vi "GenINI_Build_Read.vi"(8 "error in (no error)":errorcluster, 10 "INI read values":T1[](array[typedef]), 11 "Typedef path":path) -> (0 "error out":errorcluster, 2 "INI read values dup":T1[](array[typedef]), 3 "Typedef path dup":path)   [LabVIEW 2009]
doc: "Build an ini file reader based on the ini file information available."
uses:
  Typedefs/GenINI_Key_Values.ctl
  Typedefs/GenINI_Read_Types.ctl
  <vilib>/Utility/miscctls.llb/LVPointTypeDef.ctl
  <vilib>/Utility/miscctls.llb/LVPositionTypeDef.ctl
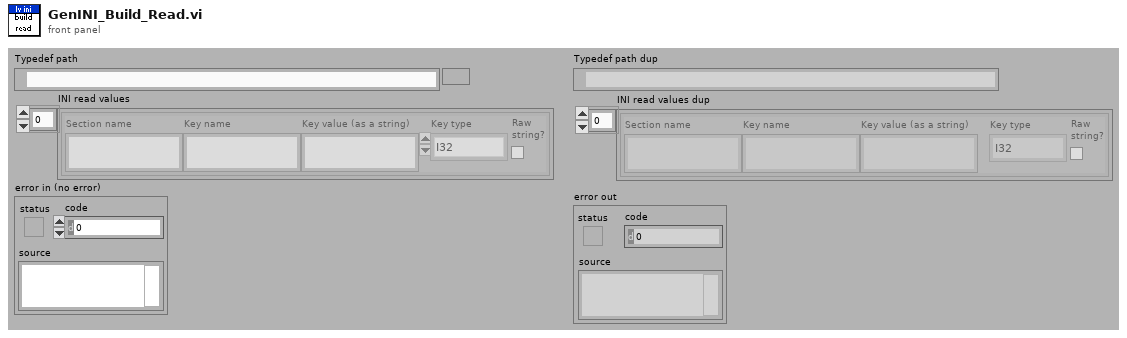
[diagram p1: front panel]
types:
  T1 = typedef "GenINI_Key_Values.ctl" = cluster{"Section name":string, "Key name":string, "Key value (as a string)":string, "Key type":T2, "Raw\nstring?":bool}
  T2 = typedef "GenINI_Read_Types.ctl" = enum16{"Boolean", "Double", "I32", "Path", "String", "U32"}
  T3 = typedef "LVPositionTypeDef.ctl" = cluster{"Left":i32, "Top":i32}
  T4 = typedef "LVPointTypeDef.ctl" = cluster{"Horizontal":i16, "Vertical":i16}
  T5 = cluster{"left":i16, "top":i16, "right":i16, "bottom":i16}
  T6 = enum32{"invalid VI type", "Standard VI", "Control VI", "Global VI", "Polymorphic VI", "Configuration VI", "SubSystem", "Facade VI", "Method VI", "Statechart Diagram VI"}
  T7 = typedef "LVRectTypeDef.ctl" = cluster{"left":i16, "top":i16, "right":i16, "bottom":i16}
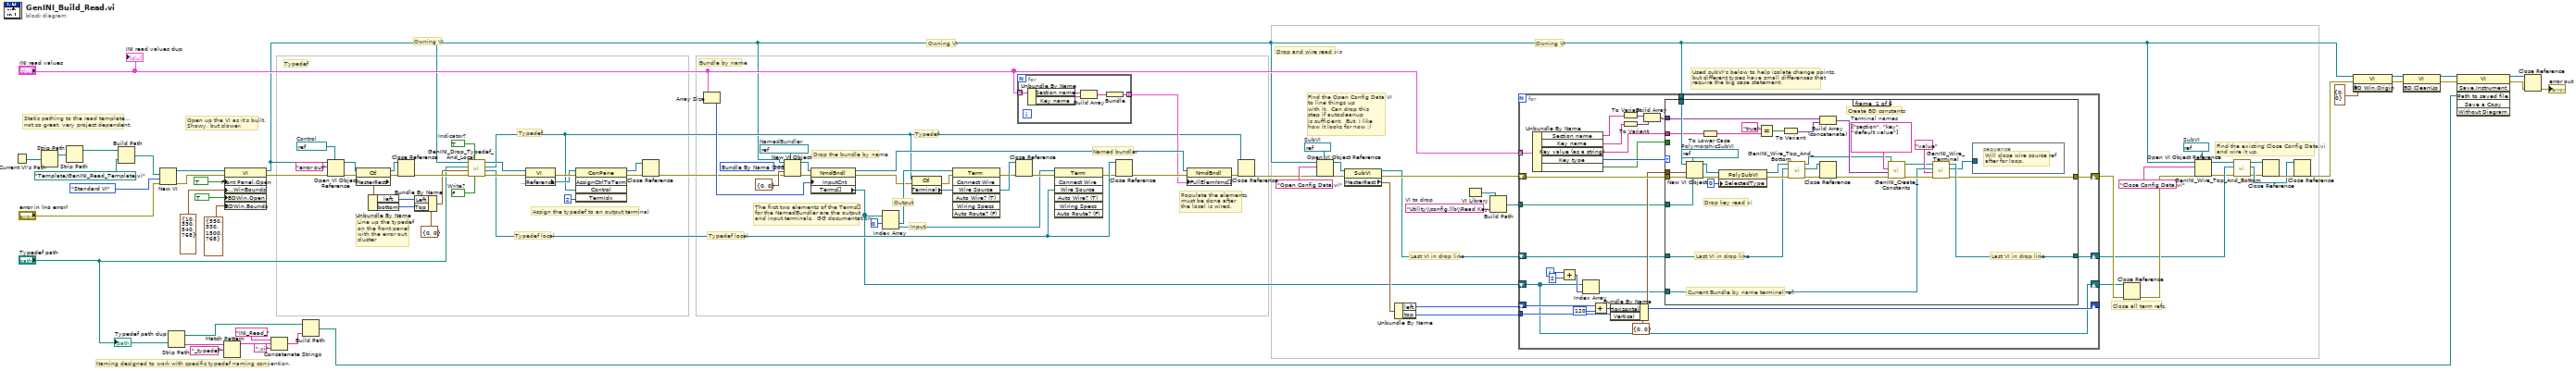
[diagram p0: block diagram]
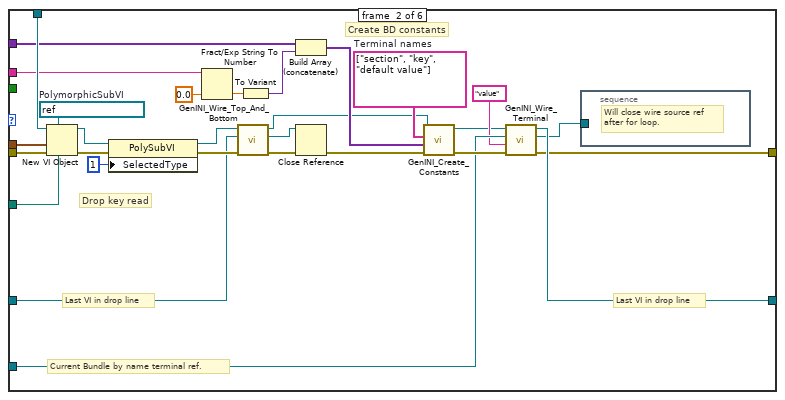
[diagram p2: hidden frame]
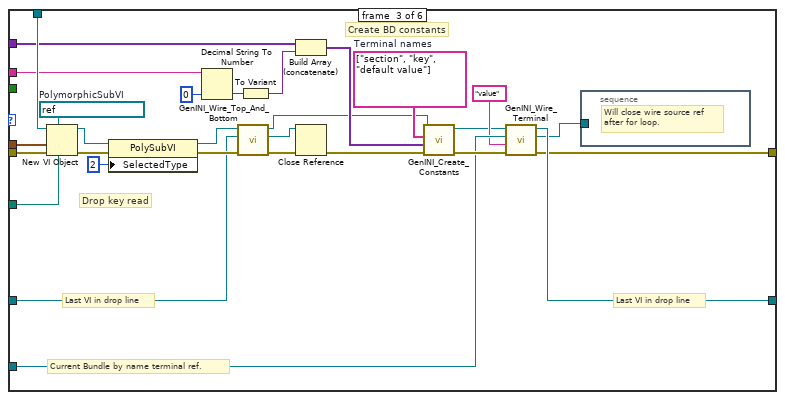
[diagram p3: hidden frame]
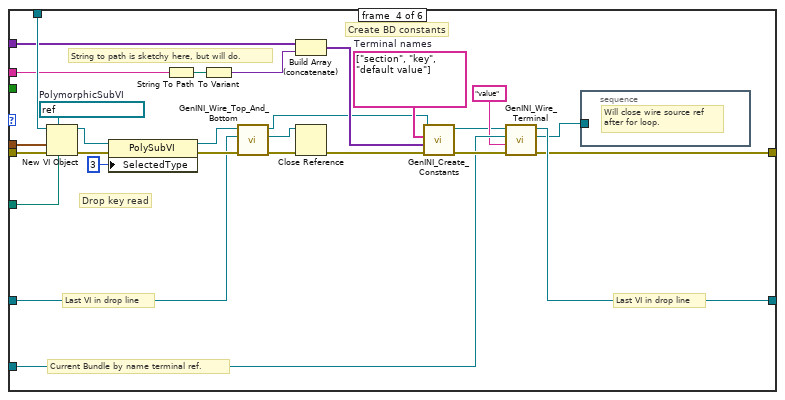
[diagram p4: hidden frame]
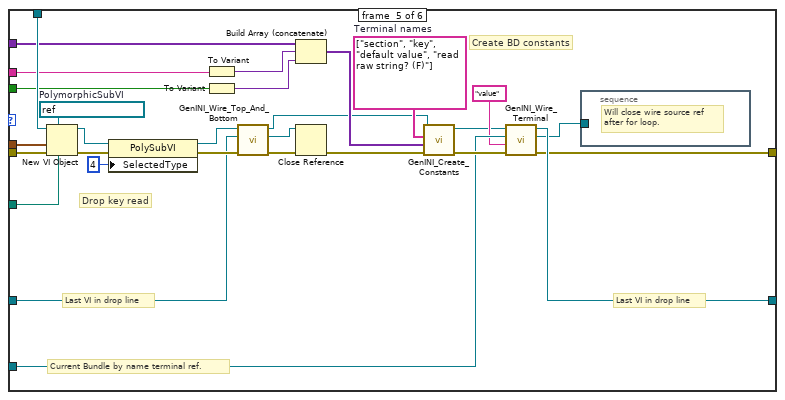
[diagram p5: hidden frame]
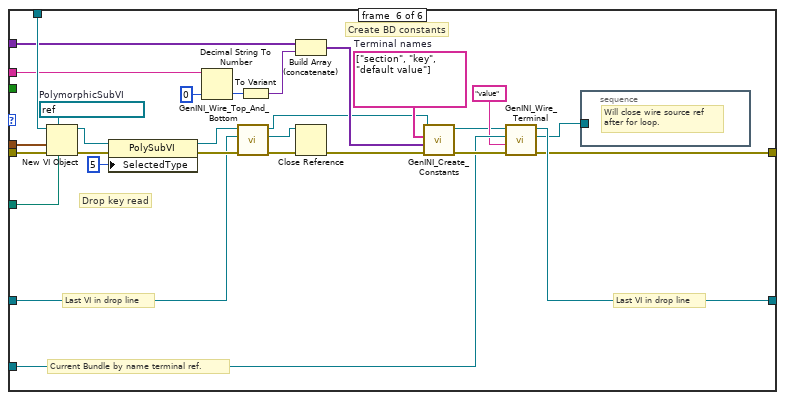
[diagram p6: hidden frame]
diagram:
  w29 = refnum<vi> refnum  # Control
  w57 = FALSE  # Write?
  w69 = TRUE  # Indicator?
  w78 = "Utility\\config.llb\\Read Key.vi"  # VI to drop
  w83 = refnum<vi> refnum  # SubVI
  w87 = refnum<vi> refnum  # SubVI
  w89 = refnum<vi> refnum  # NamedBundler
  w90 = 2057 items=[".NET Container"=2125, ".NET Refnum"=3441, "2D Picture"=3508, "3D Picture"=23776, "Absolute Value"=1054, "Access Rights"=1412, "ActiveX Container"=2072, "Add"=3915, "Add 1"=1050, "Add Array Elements"=1903, "Agitator"=3831, "AllSpoll"=1960, "Always Copy"=2400, "And"=1061, "And Array Elements"=1911, "Append True/False String"=1511, "Application Refnum"=3412, "Array"=21608, "Array 1"=3300, "Array Constant"=2070, "Array Interface Control"=23777, "Array Max & Min"=1907, "Array Size"=1809, "Array Subset"=2044, "Array To Cluster"=1168, "Array To Spreadsheet String"=1540, "Array of Strings to Path"=1422, "Atmospheric Tank"=3070, "Atmospheric Tank 1"=21751, "Automation Close"=8001, "Automation Open"=8000, "Automation Refnum"=3410, "Avogadro Constant (1/mol)"=23520, "Base 10 Logarithm Of e"=23512, "Bin"=3073, "Bin 1"=21755, "Bitpack to Array"=3135, "Blocking Variable Read"=23786, "Blocking Variable Write"=23789, "Bluetooth Close Connection"=9148, "Bluetooth Create Listener"=9151, "Bluetooth Discover"=9152, "Bluetooth Network Connection Refnum"=3468, "Bluetooth Open Connection"=9153, "Bluetooth Read"=9149, "Bluetooth Wait On Listener"=9147, "Bluetooth Write"=9150, "Boolean Array To Number"=1815, "Boolean To (0,1)"=1167, "Build Array"=2041, "Build Cluster Array"=2047, "Build Matrix"=8500, "Build Path"=1419, "Build Waveform"=2066, "Bundle"=2049, "Bundle By Name"=2057, "Byte Array To String"=1609, "Byte Stream File Refnum"=3408, "CAN Channel"=21966, "CAN Channel 1"=3340, "CAN Channel 2"=2124, "CAN Channel 3"=21817, "CAN Interface"=3339, "CAN Interface 1"=21815, "CAN Interface 2"=2123, "CAN Interface 3"=21964, "CAN Task"=3470, "CAN Task 1"=3471, "CAN Task 2"=21963, "CAN Task 3"=21789, "CPU Information"=24130, "Call By Reference Node"=3901, "Call Chain"=1999, "Call Library Function Node"=2062, "Call Parent Method"=2354, "Cancel Button"=21739, "Cancel Notification"=9107, "Carriage Return Constant"=23500, "Case Structure"=2001, "Cast Unit Bases"=1079, "Check Valve"=3833, "Checkbox"=3117, "Class Specifier Constant"=2094, "Classic Radio Buttons"=22003, "Clear Fixed-Point Overflow Status"=5562, "Close File"=1405, "Close File 1"=8052, "Close Reference"=8011, "Close Variable Connection"=23783, "Cluster"=3400, "Cluster 1"=21607, "Cluster Constant"=2071, "Cluster To Array"=1169, "Code Interface Node"=2050, "Coerce To Type"=2402, "Color Box"=3013, "Color Box Constant"=2120, "Color Box Thin Border"=2905, "Color Ramp"=3022, "Combo Box"=21604, "Combo Box 1"=3304, "Combo Box Constant"=2088, "Complex Conjugate"=1048, "Complex To Polar"=1045, "Complex To Re/Im"=1044, "Compound Arithmetic"=2200, "Compressor"=3832, "Concatenate Strings"=2040, "Conditional Disable Structure"=2064, "Constructor Node"=3904, "Control & Simulation Loop"=2099, "Control Help Window"=1353, "Control Online Help"=1355, "Control Refnum"=3419, "Convert Unit"=2059, "Conveyer"=3827, "Copy"=1416, "Copy 1"=8053, "Cosecant"=1204, "Cosine"=1201, "Cotangent"=1205, "Create Folder"=8055, "Create User Event"=2073, "Current Processor ID"=24131, "Current VI's Menubar"=9000, "Current VI's Path"=1426, "DAQmx Analog Trigger Source"=3336, "DAQmx Analog Trigger Source 1"=2119, "DAQmx Analog Trigger Source 2"=21951, "DAQmx Analog Trigger Source 3"=21774, "DAQmx Device Name"=21773, "DAQmx Device Name 1"=21950, "DAQmx Device Name 2"=2093, "DAQmx Device Name 3"=3318, "DAQmx Global Channel"=3443, "DAQmx Global Channel 1"=21770, "DAQmx Global Channel 2"=21957, "DAQmx Global Channel 3"=3430, "DAQmx Physical Channel"=3335, "DAQmx Physical Channel 1"=21954, "DAQmx Physical Channel 2"=2118, "DAQmx Physical Channel 3"=21777, "DAQmx Scale Name"=21952, "DAQmx Scale Name 1"=21775, "DAQmx Scale Name 2"=3317, "DAQmx Scale Name 3"=2116, "DAQmx Switch"=21953, "DAQmx Switch 1"=3337, "DAQmx Switch 2"=2121, "DAQmx Switch 3"=21776, "DAQmx Task Name"=3442, "DAQmx Task Name 1"=3434, "DAQmx Task Name 2"=21959, "DAQmx Task Name 3"=21778, "DAQmx Terminal"=21955, "DAQmx Terminal 1"=2117, "DAQmx Terminal 2"=21781, "DAQmx Terminal 3"=3319, "Data Cache Size"=24132, "Data Log File Refnum"=3402, "DataSocket Close"=1085, "DataSocket Open"=1084, "DataSocket Read"=1086, "DataSocket Refnum"=3417, "DataSocket Write"=1087, "Date/Time To Seconds"=1308, "Decimal Digit?"=1119, "Decimal String To Number"=1184, "Decimate 1D Array"=2046, "DecomposeArray"=2412, "DecomposeLockDataValRef"=2406, "DecomposeVariant"=2404, "Decrement"=1058, "Default Directory"=1427, "Delete"=8056, "Delete 1"=1417, "Delete Data Value Reference"=2409, "Delete From Array"=3912, "Delete Menu Items"=9004, "Delete Variant Attribute"=8206, "Delete Waveform Attribute"=8209, "Deny Access"=8057, "Dequeue Element"=9113, "Destroy User Event"=2075, "DevClear"=1961, "DevClearList"=1962, "Device Control/Status"=1433, "Device Refnum"=3405, "Diagram Disable Structure"=2054, "Dial"=3050, "Dial 1"=21732, "Digital Data"=3210, "Digital Data 1"=21216, "Digital Waveform Graph"=21718, "Digital Waveform Graph 1"=3511, "Direct Variable Read"=23785, "Direct Variable Write"=23788, "Divide"=1053, "Divide 1"=3918, "Dlg CheckBox"=21924, "Dlg Horiz Scrollbar"=21905, "Dlg Numeric"=2100, "Dlg Numeric 2"=3006, "Dlg String"=2110, "Dlg Vert Scrollbar"=21906, "Down Arrow"=3824, "Down Bow Valve"=3707, "Down Bow Valve 1"=21767, "Down Bow Valve 2"=3807, "Down Rect Valve"=21766, "Down Rect Valve 1"=3706, "Down Rect Valve 2"=3806, "Down Tee"=3818, "Down Tee 1"=3718, "EOF"=1410, "Elementary Charge (C)"=23517, "Empty Array?"=23063, "Empty Path Constant"=23523, "Empty String Constant"=23503, "Empty String/Path?"=1112, "Enable Menu Tracking"=9002, "EnableLocal"=1963, "EnableRemote"=1964, "End of Line Constant"=23525, "Enqueue Element"=9111, "Enqueue Element At Opposite End"=9129, "Enum"=3023, "Enum 1"=21605, "Enum Constant"=2090, "Equal To 0?"=1113, "Equal?"=1102, "Error Ring Constant"=2039, "Event Callback Refnum"=3435, "Event Data Node"=2102, "Event Structure"=2052, "Exchanger"=3828, "Exclusive Or"=1063, "Exponential"=1211, "Exponential (Arg) -1"=1222, "Expression Node"=2201, "FIFO Refnum"=3474, "False Constant"=2006, "Feedback Node, Feedback Node 1"=2353, "FieldPoint IO Point"=21784, "FieldPoint IO Point 1"=3440, "FieldPoint IO Point 2"=3439, "File Dialog"=8058, "File Dialog 1"=8081, "File Path Control"=21730, "File Path Control 1"=3203, "File Path Indicator"=21731, "File Path Indicator 1"=3204, "File/Directory Info"=1413, "File/Directory Info 1"=8082, "FindLstn"=1965, "FindRQS"=1966, "First Call?"=1083, "Fixed-Point Overflow?"=5565, "Fixed-Point to Integer Cast"=5566, "Flat Box"=3602, "Flat Circle"=3605, "Flat Down Triangle"=3623, "Flat Frame"=3608, "Flat Left Triangle"=3620, "Flat Right Triangle"=3621, "Flat Round Button"=3102, "Flat Rounded Box"=3611, "Flat Sequence Structure"=2069, "Flat Square Button"=3103, "Flat Up Triangle"=3622, "Flatten To String"=1164, "Flatten To XML"=8400, "Flattened String To Variant"=8202, "Floating Point Equal?"=23064, "Flush File"=8059, "Flush File 1"=1406, "Flush Queue"=9114, "For Loop"=2002, "Fork"=2194, "Format Date/Time String"=8100, "Format Into File"=2083, "Format Into String"=2081, "Format Value"=1512, "Formula Node"=2004, "Fract/Exp String To Number"=1187, "Framed Color Box"=21019, "Framed Color Box 1"=3008, "Free Label"=2321, "Furnace"=3829, "GPIB Clear"=1954, "GPIB Initialization"=1957, "GPIB Misc"=1956, "GPIB Read"=1951, "GPIB Serial Poll"=1955, "GPIB Status"=1959, "GPIB Trigger"=1953, "GPIB Wait"=1958, "GPIB Write"=1950, "Gauge"=21009, "Gauge 1"=3040, "Generate Front Panel Activity"=1329, "Generate Occurrence"=1700, "Generate User Event"=2074, "Generate User-Defined Trace Event"=2250, "Get Datalog Position"=8061, "Get Date/Time In Seconds"=1303, "Get Date/Time String"=1600, "Get Drag Drop Data"=9154, "Get File Position"=8062, "Get File Size"=8063, "Get Fixed-Point Components"=11163, "Get Help Window Status"=1354, "Get Matrix Diagonal"=8501, "Get Matrix Elements"=8502, "Get Menu Item Info"=9005, "Get Menu Selection"=9001, "Get Menu Short Cut Info"=9007, "Get Notifier Status"=9103, "Get Number of Records"=8064, "Get Permissions"=8065, "Get Queue Status"=9110, "Get Submatrix"=8503, "Get Type and Creator"=8066, "Get Variant Attribute"=8205, "Get Volume Info"=8067, "Get Waveform Attribute"=8208, "Get Waveform Components"=2067, "Global Variable"=2060, "Gravitational Constant (N m2/kg2)"=23519, "Greater Or Equal To 0?"=1114, "Greater Or Equal?"=1103, "Greater Than 0?"=1117, "Greater?"=1110, "Handle Peek"=1604, "Handle Poke"=1605, "Hex Digit?"=1123, "Hexadecimal String To Number"=1185, "Hopper"=21754, "Hopper 1"=3072, "Horiz Line"=3821, "Horiz Pipe"=3710, "Horiz Pipe 1"=3810, "Horizontal Button Box"=3636, "Horizontal Fill Slide"=3012, "Horizontal Fill Slide 1"=21100, "Horizontal Graduated Bar"=21106, "Horizontal Pointer Slide"=21101, "Horizontal Pointer Slide 1"=3011, "Horizontal Progress Bar"=21102, "Horizontal Scrollbar"=21110, "Horizontal Slide"=3010, "Horizontal Slide Switch"=3114, "Horizontal Smooth Box"=3633, "Horizontal Splitter Bar"=21861, "Horizontal Splitter Bar (Classic)"=21863, "Horizontal Splitter Bar (System)"=21865, "Horizontal Switch"=3108, "Horizontal Tank"=3071, "Horizontal Toggle Switch"=3110, "Horizontal Toggle Switch 1"=21700, "Hyperbolic Cosecant"=23053, "Hyperbolic Cosine"=1215, "Hyperbolic Cotangent"=23055, "Hyperbolic Secant"=23054, "Hyperbolic Sine"=1214, "Hyperbolic Tangent"=1216, "IMAQ Session"=3415, "IP To String"=1710, "IVI Delete Session"=8103, "IVI Logical Name"=3420, "IVI Logical Name 1"=3414, "IVI Logical Name 2"=21736, "IVI New Session"=8102, "Implies"=1080, "In Place Element Structure"=2360, "In Range and Coerce"=1127, "Include Fixed-Point Overflow Status"=5564, "Increment"=1057, "Index & Bundle Cluster Array"=2056, "Index Array"=2042, "Index String Array"=1531, "Initialize Array"=2053, "Inline C Node"=2104, "Insert Into Array"=3911, "Insert Menu Items"=9003, "Integer to Fixed-Point Cast"=5567, "Intensity Chart"=21719, "Intensity Chart 1"=3509, "Intensity Graph"=21720, "Intensity Graph 1"=3510, "Interleave 1D Arrays"=2045, "Interpolate 1D Array"=1905, "Inverse Cosecant"=23050, "Inverse Cosine"=1207, "Inverse Cotangent"=23052, "Inverse Hyperbolic Cosecant"=23056, "Inverse Hyperbolic Cosine"=1218, "Inverse Hyperbolic Cotangent"=23058, "Inverse Hyperbolic Secant"=23057, "Inverse Hyperbolic Sine"=1217, "Inverse Hyperbolic Tangent"=1219, "Inverse Secant"=23051, "Inverse Sine"=1206, "Inverse Tangent"=1208, "Inverse Tangent (2 Input)"=1228, "Invoke Node"=3900, "IrDA Close Connection"=9144, "IrDA Create Listener"=9140, "IrDA Discover"=9141, "IrDA Network Connection Refnum"=3450, "IrDA Open Connection"=9142, "IrDA Read"=9145, "IrDA Wait On Listener"=9143, "IrDA Write"=9146, "Join"=2195, "Join Numbers"=1171, "Junction"=2197, "Knob"=21000, "Knob 1"=3005, "LED Button"=3116, "LabVIEW Object"=3457, "Label"=21960, "Labeled Oblong Button"=3125, "Labeled Rectangular Button"=3124, "Labeled Round Button"=3122, "Labeled Square Button"=3123, "Leak Variant Value Reference"=2410, "Left Arrow"=3826, "Left Bow Valve"=3701, "Left Bow Valve 1"=3801, "Left Bow Valve 2"=21761, "Left Down Elbow"=3711, "Left Down Elbow 1"=3811, "Left Pump"=3713, "Left Pump 1"=3813, "Left Rect Valve"=3700, "Left Rect Valve 1"=21760, "Left Rect Valve 2"=3800, "Left Tee"=3709, "Left Tee 1"=3809, "Left Up Elbow"=3808, "Left Up Elbow 1"=3708, "Less Or Equal To 0?"=1115, "Less Or Equal?"=1104, "Less Than 0?"=1118, "Less?"=1111, "Lexical Class"=1126, "Line Feed Constant"=23501, "List Directory"=1418, "List Folder"=8083, "Listbox"=21792, "Listbox 1"=21806, "Listbox Symbol Ring Constant"=2038, "Local Variable"=2061, "Lock Range"=1411, "Logarithm Base 10"=1210, "Logarithm Base 2"=1225, "Logarithm Base X"=1224, "Logical Shift"=1081, "Lossy Enqueue Element"=9130, "Lowered Rounded Box"=3638, "MATLAB script"=9020, "Machine Epsilon"=23528, "MakeAddr"=1967, "Mantissa & Exponent"=1150, "Match First String"=1532, "Match Pattern"=1535, "Match True/False String"=1533, "MathScript Call By Reference Node"=3906, "MathScript Node"=2357, "Matrix Size"=8507, "Max & Min"=1108, "Menu Refnum"=3413, "Menu Ring"=3018, "Menu Ring 1"=21600, "Menu-Popup Ring"=3017, "Merge Signals"=2350, "Meter"=21008, "Meter 1"=3030, "Mixed Signal Graph"=21721, "Molar Gas Constant (J/(mol K))"=23522, "Motion Resource"=21787, "Motion Resource 1"=3448, "Motion Resource 2"=3449, "Motor"=3720, "Motor 1"=3820, "Move"=1415, "Move 1"=8068, "Multi-Segment Pipe"=23780, "Multicolumn Listbox"=21799, "Multicolumn Listbox 1"=21791, "Multiple Selection Listbox"=3208, "Multiply"=1052, "Multiply 1"=3917, "Multiply Array Elements"=1904, "Multirate Structure"=2199, "Natural Logarithm"=1209, "Natural Logarithm (Arg +1)"=1221, "Natural Logarithm Base"=23510, "Natural Logarithm Of 10"=23513, "Natural Logarithm Of 2"=23514, "Natural Logarithm Of Pi"=23508, "Negate"=1069, "Negative Infinity"=23509, "New Data Value Reference"=2408, "New Directory"=1402, "New File"=1404, "New VI"=8014, "New VI Object"=8015, "Not"=1064, "Not A Number/Path/Refnum?"=1128, "Not A Path Constant"=23524, "Not And"=1071, "Not Equal To 0?"=1116, "Not Equal?"=1105, "Not Exclusive Or"=1073, "Not Or"=1072, "Not a Refnum Constant"=23526, "Not a Shared Variable"=23527, "Notifier Refnum"=3423, "Number To Boolean Array"=1814, "Number To Decimal String"=1180, "Number To Engineering String"=1183, "Number To Exponential String"=1505, "Number To Fractional String"=1506, "Number To Hexadecimal String"=1181, "Number To Octal String"=1182, "Number of Cache Levels"=24133, "Numeric Constant"=2005, "Numeric Control"=3000, "Numeric Control 1"=21003, "Numeric Indicator"=3001, "Numeric Indicator 1"=21004, "OK Button"=21738, "OLE Variant"=3150, "Obtain Notifier"=9101, "Obtain Queue"=9108, "Occurrence Refnum"=3406, "Octal Digit?"=1129, "Octal String To Number"=1186, "Old VISA Open"=1921, "One Button Dialog"=1340, "Open Application Reference"=8012, "Open Device"=1430, "Open File"=1403, "Open Tank"=21752, "Open Tank 1"=3074, "Open VI Object Reference"=8013, "Open VI Reference"=8010, "Open Variable Connection"=23779, "Open Variable Connection in Background"=23791, "Open and Verify Variable Connection"=23790, "Open/Create/Replace Datalog"=8054, "Open/Create/Replace File"=8050, "Or"=1062, "Or Array Elements"=1910, "PPoll"=1969, "PPollConfig"=1970, "PPollUnconfig"=1971, "Package Matrix"=23001, "PassControl"=1968, "Path Constant"=2009, "Path To String"=1077, "Path Type"=1421, "Path to Array of Strings"=1423, "Pi"=23504, "Pi Divided By 2"=23506, "Pi Multiplied By 2"=23505, "Pick Line"=1510, "Pict Ring"=21602, "Pict Ring 1"=3015, "PixMap"=3505, "PixMap (Do not touch it!!)"=3507, "Planck's Constant (J/Hz)"=23516, "Platform Flat Square Button"=3134, "Plug-In Control"=21820, "Polar To Complex"=1047, "Polar To Re/Im"=23061, "Positive Infinity"=23515, "Power Of 10"=1212, "Power Of 2"=1223, "Power Of X"=1213, "Preserve Run-Time Class"=8018, "Pressure Tank"=3075, "Pressure Tank 1"=21753, "Preview Queue Element"=9112, "Printable?"=1124, "Property Node"=1920, "Pulldown Menu Ring"=3061, "Push Button"=21001, "Queue Refnum"=3424, "Quit LabVIEW"=1352, "Quotient & Remainder"=1056, "RT FIFO Create"=24000, "RT FIFO Delete"=24003, "RT FIFO Read"=24001, "RT FIFO Write"=24002, "Radio Buttons"=22001, "Raised Box"=3600, "Raised Box 1"=3637, "Raised Circle"=3603, "Raised Down Triangle"=3615, "Raised Frame"=3606, "Raised Left Triangle"=3612, "Raised Right Triangle"=3613, "Raised Rounded Box"=3609, "Raised Up Triangle"=3614, "Random Number (0-1)"=1070, "RcvRespMsg"=1972, "Re/Im To Complex"=1046, "Re/Im To Polar"=23060, "Read Datalog"=8069, "Read Device"=1432, "Read File"=1407, "Read Variable"=23781, "Read from Binary File"=8051, "Read from Text File"=8070, "ReadStatus"=1973, "Receive"=1974, "ReceiveSetup"=1975, "Recessed Box"=3601, "Recessed Circle"=3604, "Recessed Down Triangle"=3619, "Recessed Frame"=3607, "Recessed Left Triangle"=3616, "Recessed Menu Ring"=3019, "Recessed Right Triangle"=3617, "Recessed Rounded Box"=3610, "Recessed Up Triangle"=3618, "Reciprocal"=1059, "Reciprocal Of Pi"=23507, "Reciprocal Of e"=23511, "RecomposeArray"=2403, "RecomposeUnlockDataValRef"=2407, "RecomposeVariant"=2405, "Rectangular Stop Button"=3128, "Refnum to Path"=1424, "Refnum to Session"=2306, "Region"=2196, "Register Event Callback"=2078, "Register For Events"=2065, "Register Session"=2319, "Release Notifier"=9102, "Release Queue"=9109, "Remove Fixed-Point Overflow Status"=5563, "Replace Array Subset"=3910, "Replace Substring"=3913, "Request Deallocation"=1610, "ResetSys"=1976, "Reshape Array"=2055, "Resize Matrix"=8508, "Reverse 1D Array"=1900, "Reverse String"=1537, "Right Arrow"=3825, "Right Bow Valve"=21765, "Right Bow Valve 1"=3705, "Right Bow Valve 2"=3805, "Right Down Elbow"=3817, "Right Down Elbow 1"=3717, "Right Pump"=3719, "Right Pump 1"=3819, "Right Rect Valve"=3804, "Right Rect Valve 1"=3704, "Right Rect Valve 2"=21764, "Right Tee"=3715, "Right Tee 1"=3815, "Right Up Elbow"=3814, "Right Up Elbow 1"=3714, "Ring Constant"=2008, "Rocker"=21002, "Rotary Feeder"=3830, "Rotate"=1082, "Rotate 1D Array"=1906, "Rotate Left With Carry"=1606, "Rotate Right With Carry"=1607, "Rotate String"=1536, "Round Button"=3100, "Round LED"=3120, "Round LED 1"=21012, "Round Light"=3104, "Round Push Button"=3112, "Round Push Button 2"=3118, "Round Radio Button"=3106, "Round Stop Button"=3127, "Round To Nearest"=1055, "Round Toward +Infinity"=1076, "Round Toward -Infinity"=1075, "Rydberg Constant (1/m)"=23521, "Scale By Power Of 2"=1074, "Scan From File"=2082, "Scan From String"=2080, "Scan String For Tokens"=8101, "Scan Value"=1534, "Scanned Variable Read"=23784, "Scanned Variable Write"=23787, "Search 1D Array"=1901, "Search and Replace String"=3914, "Search/Split String"=1538, "Secant"=1203, "Seconds To Date/Time"=1309, "Seek"=1409, "Select"=1516, "Send"=1977, "Send Notification"=9104, "SendCmds"=1978, "SendDataBytes"=1979, "SendIFC"=1980, "SendLLO"=1982, "SendList"=1981, "SendSetup"=1983, "Session to Refnum"=2307, "Set Datalog Position"=8072, "Set File Position"=8073, "Set File Size"=8074, "Set Matrix Diagonal"=8504, "Set Matrix Elements"=8505, "Set Menu Item Info"=9006, "Set Number of Records"=8075, "Set Occurrence"=1702, "Set Permissions"=8076, "Set Submatrix"=8506, "Set Type and Creator"=8077, "Set Variant Attribute"=8204, "Set Waveform Attribute"=8207, "SetRWLS"=1984, "SetTimeOut"=1985, "Shared Variable"=23778, "Shared Variable Constant"=3473, "Shared Variable Control"=3472, "Shared Variable Control 1"=21814, "Shared Variable to String"=1831, "Sign"=1049, "Simple Horizontal Slide"=3003, "Simple Numeric"=3029, "Simple Numeric 1"=2900, "Simple String"=2115, "Simple Vertical Slide"=3002, "Sinc"=1227, "Sine"=1200, "Sine & Cosine"=1220, "Size Handle"=1603, "Slide Switch"=21011, "Sort 1D Array"=1120, "Sort Array of String, Sort Array of String 1"=23065, "Speed Of Light In Vacuum (m/sec)"=23518, "Split 1D Array"=1908, "Split Button"=21020, "Split Number"=1170, "Split Signals"=2351, "Spreadsheet String To Array"=1539, "Square"=23059, "Square Button"=3101, "Square LED"=3121, "Square LED 1"=21013, "Square Light"=3105, "Square Push Button"=3113, "Square Push Button 2"=3119, "Square Radio Button"=3107, "Square Root"=1060, "Stacked Sequence Structure"=2000, "State"=2198, "State Diagram"=2051, "Static VI Reference"=2084, "Stop"=1350, "Stop Button"=21230, "String Constant"=2007, "String Control"=3200, "String Control 1"=21701, "String Indicator"=3201, "String Indicator 1"=21702, "String Length"=1502, "String Subset"=1503, "String To Byte Array"=1608, "String To IP"=1711, "String To Path"=1078, "String to Shared Variable"=1830, "Strip Path"=1420, "SubPanel"=21810, "SubPanel (Classic)"=21811, "SubPanel (System)"=21823, "Subtract"=1051, "Subtract 1"=3916, "Swap Bytes"=1162, "Swap Values"=2401, "Swap Vector Element"=1912, "Swap Words"=1163, "System Button"=3130, "System Cancel Button"=3131, "System Checkbox"=3132, "System Chiseled Line"=3632, "System Colored Rectangle"=3625, "System Combo Box"=21917, "System Enum"=3062, "System Horizontal Pointer Slide"=21902, "System Horizontal Progress Bar"=21910, "System Horizontal Slide"=21904, "System Label"=21961, "System Listbox"=21805, "System Mixed Checkbox"=21333, "System Multicolumn Listbox"=21798, "System Numeric"=21919, "System Path Control"=21922, "System Pict Ring"=21925, "System Radio Button"=3133, "System Radio Buttons"=22002, "System Recessed Frame"=3624, "System Ring"=3060, "System Spin Control"=21900, "System String"=21920, "System Tab Control"=3331, "System Table"=21797, "System Time Stamp"=21967, "System Tree"=21794, "System Vertical Pointer Slide"=21901, "System Vertical Progress Bar"=21909, "System Vertical Slide"=21903, "TCP Close Connection"=1713, "TCP Create Listener"=1717, "TCP Flattened Read"=1718, "TCP Flattened Write"=1719, "TCP Flex Read"=1720, "TCP Flex Write"=1721, "TCP Network Connection Refnum"=3407, "TCP Open Connection"=1715, "TCP Read"=1716, "TCP Wait On Listener"=1712, "TCP Write"=1714, "TDMS Close"=24113, "TDMS Defragment"=24119, "TDMS File"=3477, "TDMS Flush"=24117, "TDMS Get Properties"=24115, "TDMS List Contents"=24116, "TDMS Open"=24112, "TDMS Read"=24111, "TDMS Refnum To File ID"=24120, "TDMS Set Properties"=24114, "TDMS Write"=24110, "TDMS Write IP"=24118, "Tab Constant"=23502, "Tab Control"=3330, "Tab Control 1"=3332, "Table"=21796, "Table 1"=21790, "Tag Attribute Ring"=2063, "Tangent"=1202, "Tank"=21006, "Tank 1"=3020, "Temporary Directory"=1435, "TestSRQ"=1986, "TestSys"=1987, "Text & Pict Ring"=21603, "Text & Pict Ring 1"=3016, "Text Button"=21015, "Text Ring"=21601, "Text Ring 1"=3014, "Text to UTF-8"=23066, "Thermometer"=21007, "Thermometer 1"=3021, "Thick Chiseled Line"=3630, "Thick Line"=3629, "Thick Line with Arrow"=3631, "Thick Lowered Box"=3635, "Thin Chiseled Line"=3627, "Thin Line"=3626, "Thin Line with Arrow"=3628, "Threshold 1D Array"=1909, "Tick Count (ms)"=1300, "Time Stamp Constant"=2068, "Time Stamp Control"=21913, "Time Stamp Control 1"=5555, "Time Stamp Indicator"=21914, "Time Stamp Indicator 1"=5556, "Timed Loop"=5570, "Timed Sequence"=5573, "To Byte Integer"=1140, "To Double Precision Complex"=1152, "To Double Precision Float"=1147, "To Extended Precision Complex"=1154, "To Extended Precision Float"=1149, "To Fixed-Point"=5561, "To Long Integer"=1142, "To Lower Case"=1189, "To More Generic Class"=8017, "To More Specific Class"=8016, "To OLE Variant"=8002, "To Probe String"=2413, "To Quad Integer"=1155, "To Single Precision Complex"=1151, "To Single Precision Float"=1146, "To Time Stamp"=5560, "To Unsigned Byte Integer"=1143, "To Unsigned Long Integer"=1145, "To Unsigned Quad Integer"=1156, "To Unsigned Word Integer"=1144, "To Upper Case"=1188, "To Variant"=8201, "To Word Integer"=1141, "Traditional DAQ Channel"=21733, "Traditional DAQ Channel 1"=2085, "Traditional DAQ Channel 2"=3320, "Transpose 1D Array"=23068, "Transpose 2D Array"=1902, "Transpose Matrix"=8509, "Tree"=21819, "Tree 1"=21793, "Trigger"=1988, "TriggerList"=1989, "Two Button Dialog"=1341, "Type Cast"=1166, "Type and Creator"=1434, "UDP Close"=1726, "UDP Multicast Open"=1727, "UDP Network Connection Refnum"=3418, "UDP Open"=1723, "UDP Read"=1724, "UDP Write"=1725, "UTF-8 to Text"=23067, "Unbitpack from Array"=3136, "Unbundle"=2048, "Unbundle By Name"=2058, "Unflatten From String"=1165, "Unflatten From XML"=8401, "Unleak Variant Value Reference"=2411, "Unpackage Matrix"=23000, "Unregister For Events"=2076, "Unregister Session"=2320, "Up Arrow"=3823, "Up Bow Valve"=3703, "Up Bow Valve 1"=3803, "Up Bow Valve 2"=21763, "Up Rect Valve"=3702, "Up Rect Valve 1"=21762, "Up Rect Valve 2"=3802, "Up Tee"=3712, "Up Tee 1"=3812, "User Defined Refnum"=3428, "User Defined Refnum Tag"=21745, "User Defined Refnum Tag 1"=3429, "User Defined Refnum Tag Constant"=3426, "User Defined Refnum Tag Flatten"=21747, "User Defined Refnum Tag Flatten 1"=3454, "User Defined Tag"=21749, "User Defined Tag 1"=3329, "User Defined Tag Constant"=2114, "User Item"=3506, "VI Library"=1425, "VI Refnum"=3422, "VI Server Reference"=2091, "VISA Assert Interrupt Signal"=2309, "VISA Assert Trigger"=1929, "VISA Assert Utility Signal"=2310, "VISA Clear"=1927, "VISA Close"=1922, "VISA Disable Event"=1940, "VISA Discard Events"=1941, "VISA Enable Event"=1942, "VISA Find Resource"=1923, "VISA Flush I/O Buffer"=2302, "VISA GPIB Command"=2315, "VISA GPIB Control ATN"=2316, "VISA GPIB Control REN"=2304, "VISA GPIB Pass Control"=2317, "VISA GPIB Send IFC"=2318, "VISA In 16"=1930, "VISA In 32"=1944, "VISA In 64"=2140, "VISA In 8"=1936, "VISA Lock"=1993, "VISA Map Address"=1932, "VISA Map Trigger"=2311, "VISA Memory Allocation"=1997, "VISA Memory Allocation Ex"=2146, "VISA Memory Free"=1998, "VISA Move"=2303, "VISA Move In 16"=1948, "VISA Move In 32"=1991, "VISA Move In 64"=2144, "VISA Move In 8"=1946, "VISA Move Out 16"=1949, "VISA Move Out 32"=1992, "VISA Move Out 64"=2145, "VISA Move Out 8"=1947, "VISA Open"=2308, "VISA Out 16"=1931, "VISA Out 32"=1945, "VISA Out 64"=2141, "VISA Out 8"=1937, "VISA Peek 16"=1934, "VISA Peek 32"=1995, "VISA Peek 64"=2142, "VISA Peek 8"=1938, "VISA Poke 16"=1935, "VISA Poke 32"=1996, "VISA Poke 64"=2143, "VISA Poke 8"=1939, "VISA Read"=1925, "VISA Read STB"=1928, "VISA Read To File"=2313, "VISA Refnum to Session"=2300, "VISA Resource Name"=3421, "VISA Set I/O Buffer Size"=2301, "VISA Status Description"=1924, "VISA USB Control In"=2086, "VISA USB Control Out"=2087, "VISA Unlock"=1994, "VISA Unmap Address"=1933, "VISA Unmap Trigger"=2312, "VISA VXI Cmd or Query"=2305, "VISA Wait on Event"=1943, "VISA Write"=1926, "VISA Write From File"=2314, "VISA resource name"=3409, "VISA resource name 1"=21737, "Variable Class Specifier Constant"=2106, "Variable Configuration"=3475, "Variant"=3310, "Variant To Data"=8003, "Variant To Flattened String"=8203, "Vert Line"=3822, "Vert Pipe"=3816, "Vert Pipe 1"=3716, "Vert Rocker"=21740, "Vertical Fill Slide"=21014, "Vertical Fill Slide 1"=3009, "Vertical Graduated Bar"=21107, "Vertical Pointer Slide"=21017, "Vertical Pointer Slide 1"=3007, "Vertical Progress Bar"=21104, "Vertical Scrollbar"=21111, "Vertical Slide"=3004, "Vertical Slide Switch"=21741, "Vertical Slide Switch 1"=3115, "Vertical Smooth Box"=3634, "Vertical Splitter Bar"=21860, "Vertical Splitter Bar (Classic)"=21862, "Vertical Splitter Bar (System)"=21864, "Vertical Switch"=3109, "Vertical Toggle Switch"=21005, "Vertical Toggle Switch 1"=3111, "Volume Info"=1414, "Wait (ms)"=1302, "Wait For Activity"=1722, "Wait For Front Panel Activity"=1328, "Wait Until Next ms Multiple"=1327, "Wait for GPIB RQS"=1952, "Wait on Notification"=9105, "Wait on Notification from Multiple"=9106, "Wait on Notification from Multiple with Notifier History"=9132, "Wait on Notification with Notifier History"=9131, "Wait on Occurrence"=1701, "WaitSRQ"=1990, "Waveform Chart"=21010, "Waveform Chart 1"=3501, "Waveform Chart 2"=21717, "Waveform Graph"=21703, "Waveform Graph 1"=3504, "While Loop"=2003, "While Loop 1"=2352, "White Space?"=1125, "Write Datalog"=8079, "Write Device"=1431, "Write File"=1408, "Write Variable"=23782, "Write to Binary File"=8078, "Write to Text File"=8080, "XY Graph"=21716, "XY Graph 1"=3500, "Y-th Root of X"=23062]
  # "Naming designed to work with specific typedef naming convention."
  # "Line up the typedef\non the front panel\nwith the error out\ncluster"
  # "Typedef"
  # "Typedef local"
  # "Owning VI"
  # "Used subVI's below to help isolate change points,\nbut different types have small differences that\nrequire the big case statement."
  # "Owning VI"
  # "Close all term refs."
  # "Drop and wire read vis"
  # "Typedef local"
  # "Last VI in drop line"
  # "Typedef"
  # "Bundle by name"
  # "Named bundler"
  # "Input"
  # "The first two elements of the Terms[]\nfor the NamedBundler are the output\nand input terminals.  GG documentation."
  # "Drop the bundle by name"
  # "Typedef"
  # "Owning VI"
  # "Open up the VI as it's built.\nShowy, but slower."
  # "Static pathing to the read template...\nnot so great, very project dependent."
  # "Populate the elements,\nmust be done after\nthe local is wired."
  # "Output"
  # "Assign the typedef to an output terminal"
  # "Find the Open Config Data VI\nto line things up\nwith it.  Can drop this\nstep if autocleanup\nis sufficient.  But, I like\nhow it looks for now :)"
  # "Find the existing Close Config Data.vi\nand wire it up."
  n1 = Current VI's Path() -> (path=w96:path)
  n2 = Strip Path(path=w96) -> (stripped path=w95:path)  [unwired: 1 out]
  n3 = Strip Path(path=w95) -> (stripped path=w94:path)  [unwired: 1 out]
  n4 = Build Path(base path=w94, name or relative path=path "Template/GenINI_Read_Template.vi") -> (appended path=w97:path)
  n5 = New VI(8:"error in (no error)", 9:T6."Standard VI" ("vi type (standard vi)"), 10:w97) -> (0:w100:errorcluster, 3:w102:refnum<vi>)  [unwired: 4 in]
  n6 = Strip Path(path="Typedef path") -> (stripped path=w6:path, name=w11:string)
  n7 = Match Pattern(string=w11, regular expression="_typedef") -> (before substring=w10:string)  [unwired: 1 in, 3 out]
  n8 = property class="VI"(reference=w102, error in=w100, "Front Panel.Open"=TRUE ("Front Panel Window:Open"), "Front Panel.WinBounds"=T5 {"left"=10, "top"=330, "right"=540, "bottom"=768} ("Block Diagram Window:Window Bounds"), "BDWin.Open"=TRUE ("Block Diagram Window:Open"), "BDWin.Bounds"=T5 {"left"=550, "top"=330, "right"=1500, "bottom"=768} ("Block Diagram Window:Window Bounds")) -> (reference out=w18:refnum<vi>, error out=w20:errorcluster)
  n9 = Concatenate Strings("INI_Read_", w10, ".vi" ("string")) -> (w7:string)
  n10 = Build Path(base path=w6, name or relative path=w7) -> (appended path=w5:path)
  n11 = Open VI Object Reference(7:w29, 8:w20, 10:"error out" ("name/order"), 11:w18) -> (0:w27:errorcluster, 3:w26:refnum<vi>)
  n12 = property class="Ctl"(reference=w26, error in=w27) -> (reference out=w25:refnum<vi>, error out=w22:errorcluster, "MasterRect"=w23:T7)
  n13 = Unbundle By Name(w23) -> ("left"=w16:i16, "bottom"=w15:i16)
  n14 = Close Reference(reference=w25, error in (no error)=w22) -> (error out=w19:errorcluster)
  n15 = Bundle By Name(cluster=T3 {"Left"=0, "Top"=0} ("Position"), "Left"=w16, "Top"=w15) -> (w14:T3)
  n16 = call "GenINI_Drop_Typedef_And_Local.vi"("Local is write? (F)"=w57, "Typedef is indicator? (F)"=w69, "error in"=w19, "Location (0,0)"=w14, "Typedef path"="Typedef path", "owning vi ref"=w18) -> ("error out"=w56:errorcluster, "typedef local ref"=w52:refnum<vi>, "typedef ref"=w24:refnum<vi>, "owning vi ref dup"=w30:refnum<vi>)  [unwired: 2 in]
  n17 = property class="VI"(reference=w30, error in=w56) -> (error out=w68:errorcluster, "Connector Pane:Reference"=w37:refnum<vi>)  [unwired: 1 out]
  n18 = invoke class="ConPane" method="AssignCtrlToTerm"(reference=w37, error in=w68, "Control"=w24, "TermIdx"=u32 2 ("Terminal Index")) -> (reference out=w64:refnum<vi>, error out=w66:errorcluster)  [unwired: 1 in, 3 out]
  n19 = Close Reference(reference=w64, error in (no error)=w66) -> (error out=w21:errorcluster)
  n20 = Array Size(array="INI read values") -> (size(s)=w51:i32)
  n21 = New VI Object(vi object class=w89, owner refnum=w18, style=w90, position/next to=T4 {"Horizontal"=0, "Vertical"=0} ("relative position/next to refnum"), 8:w21) -> (object refnum=w61:refnum<vi>, 0:w62:errorcluster)  [unwired: 3 in]
  n22 = property class="NmdBndl"(reference=w61, error in=w62, "InputCnt"=w51) -> (reference out=w48:refnum<vi>, error out=w50:errorcluster, "Terms[]"=w42:refnum<vi>[])
  n23 = Index Array(array=w42, index #1=0 ("index")) -> (element #1=w59:refnum<vi>, element #2=w53:refnum<vi>)  [unwired: 1 in]
  n24 = property class="Ctl"(reference=w24, error in=w50) -> (error out=w58:errorcluster, "Terminal"=w55:refnum<vi>)  [unwired: 1 out]
  n25 = invoke class="Term" method="Connect Wire"(reference=w59, error in=w58, "Wire Source"=w55) -> (error out=w45:errorcluster)  [unwired: 4 in, 6 out]
  n26 = Close Reference(reference=w55, error in (no error)=w45) -> (error out=w54:errorcluster)
  n27 = for {
    tunnel: "INI read values" -> [w108] mode=indexing
    tunnel: [w104] -> w46 mode=indexing
    n28 = Unbundle By Name(w108) -> ("Section name"=w107:string, "Key name"=w106:string)
    n29 = Build Array(w107, w106) -> (w105:string[])
    n30 = Bundle(w105) -> (w104:cluster{string[]})  [unwired: 1 in]
  }
  n31 = invoke class="Term" method="Connect Wire"(reference=w53, error in=w54, "Wire Source"=w52) -> (error out=w43:errorcluster)  [unwired: 4 in, 6 out]
  n32 = Close Reference(reference=w52, error in (no error)=w43) -> (error out=w49:errorcluster)
  n33 = property class="NmdBndl"(reference=w48, error in=w49, "FullElemNms[]"=w46) -> (error out=w44:errorcluster)  [unwired: 1 out]
  n34 = Close Reference(reference=w24, error in (no error)=w44) -> (error out=w65:errorcluster)
  n35 = Open VI Object Reference(7:w83, 8:w65, 10:"Open Config Data.vi" ("name/order"), 11:w18) -> (0:w84:errorcluster, 3:w85:refnum<vi>)
  n36 = property class="SubVI"(reference=w85, error in=w84) -> (reference out=w72:refnum<vi>, error out=w73:errorcluster, "MasterRect"=w81:T7)
  n37 = Unbundle By Name(w81) -> ("left"=w80:i16, "top"=w79:i16)
  n38 = VI Library() -> (path=w77:path)
  n39 = Build Path(base path=w77, name or relative path=w78) -> (appended path=w76:path)
  n40 = for {
    tunnel: w18 -> [w133]
    tunnel: w79 -> [w128]
    shift-right: [w127] -> _
    shift-left: w80 -> [w131]
    tunnel: "INI read values" -> [w126] mode=indexing
    tunnel: w76 -> [w124]
    shift-right: [w115] -> w41
    shift-left: w73 -> [w134]
    shift-right: [w116] -> w35
    shift-left: w72 -> [w117]
    shift-right: [w110] -> w39
    shift-left: w42 -> [w110]
    i -> [w114]
    n41 = Unbundle By Name(w126) -> ("Section name"=w123:string, "Key name"=w122:string, "Key value (as a string)"=w118:string, "Key type"=w125:T2, "Raw\nstring?"=w109:bool)
    n42 = Add(x=w114, y=2) -> (x+y=w112:i32)
    n43 = Index Array(array=w110, index=w112) -> (element=w111:refnum<vi>)
    n44 = Add(x=w131, y=i16 120) -> (x+y=w127:i16)
    n45 = Bundle By Name(cluster=T4 {"Horizontal"=0, "Vertical"=0} ("relative position/next to refnum"), "Horizontal"=w127, "Vertical"=w128) -> (w129:T4)
    n46 = To Variant(anything=w123) -> (Variant=w121:variant)
    n47 = To Variant(anything=w122) -> (Variant=w120:variant)
    n48 = Build Array(w121, w120) -> (w119:variant[])
    n49 = case shown="\"Boolean\"" w125 {
      tunnel: w134 -> [w160 w189 w218 w246 w275 w304]
      tunnel: w133 -> [w159 w188 w217 w245 w274 w303]
      tunnel: w129 -> [w158 w187 w216 w244 w273 w302]
      tunnel: w124 -> [w157 w186 w215 w243 w272 w301]
      tunnel: w119 -> [w155 w184 w213 w241 w270 w299]
      tunnel: w118 -> [w138 w182 w211 w225 w253 w297]
      tunnel: w117 -> [w150 w176 w205 w236 w264 w291]
      tunnel: [w144 w170 w199 w230 w258 w285] -> w116
      tunnel: [w141 w167 w196 w227 w255 w282] -> w115
      tunnel: w111 -> [w147 w173 w202 w233 w261 w288]
      tunnel: w109 -> [_ _ _ _ w252 _]
      frame #0 {
        w156 = string[] ["section", "key", "default value"]  # Terminal names
        w164 = refnum<vi> refnum  # PolymorphicSubVI
        # "Last VI in drop line"
        # "Last VI in drop line"
        # "Current Bundle by name terminal ref."
        # "Drop key read vi"
        # "Create BD constants"
        n50 = New VI Object(vi object class=w164, owner refnum=w159, position/next to=w158, 6:w157, 8:w160) -> (object refnum=w163:refnum<vi>, 0:w161:errorcluster)  [unwired: 3 in]
        n51 = To Lower Case(string=w138) -> (all lower case string=w137:string)
        n52 = property class="PolySubVI"(reference=w163, error in=w161, "SelectedType"=0 ("Selected Type")) -> (reference out=w153:refnum<vi>, error out=w151:errorcluster)
        n53 = Equal?(x="true", y=w137) -> (x = y?=w136:bool)
        n54 = To Variant(anything=w136) -> (Variant=w135:variant)
        n55 = call "GenINI_Wire_Top_And_Bottom.vi"("error in"=w151, "vi 2 ref"=w150, "vi 1 ref"=w153) -> ("error out"=w143:errorcluster, "vi 2 ref dup"=w149:refnum<vi>, "vi 1 ref dup"=w152:refnum<vi>)  [unwired: 6 in]
        n56 = Build Array (concatenate)(w155, w135) -> (w154:variant[])
        n57 = Close Reference(reference=w149, error in (no error)=w143) -> (error out=w142:errorcluster)
        n58 = call "GenINI_Create_Constants.vi"("error in"=w142, "Data array"=w154, "Terminal names"=w156, "vi ref"=w152) -> ("error out"=w148:errorcluster, "vi ref dup"=w145:refnum<vi>)  [unwired: 6 in]
        n59 = call "GenINI_Wire_Terminal.vi"("error in"=w148, "Terminal  name"="value", "Wire source ref"=w147, "vi ref"=w145) -> ("error out"=w141:errorcluster, "Wire source ref dup"=w140:refnum<vi>, "vi ref dup"=w144:refnum<vi>)  [unwired: 5 in]
        n60 = stacked-sequence {
          tunnel: w140 -> [_]
          frame #0 {
            # "Will close wire source ref\nafter for loop."
          }
        }
      }
      frame #1 {
        w185 = string[] ["section", "key", "default value"]  # Terminal names
        w193 = refnum<vi> refnum  # PolymorphicSubVI
        # "Last VI in drop line"
        # "Last VI in drop line"
        # "Current Bundle by name terminal ref."
        # "Drop key read"
        # "Create BD constants"
        n61 = New VI Object(vi object class=w193, owner refnum=w188, position/next to=w187, 6:w186, 8:w189) -> (object refnum=w192:refnum<vi>, 0:w190:errorcluster)  [unwired: 3 in]
        n62 = property class="PolySubVI"(reference=w192, error in=w190, "SelectedType"=1 ("Selected Type")) -> (reference out=w179:refnum<vi>, error out=w177:errorcluster)
        n63 = Fract/Exp String To Number(string=w182, default (0 dbl)=0.0 ("default (0 I32)")) -> (number=w181:dbl)  [unwired: 2 in, 1 out]
        n64 = call "GenINI_Wire_Top_And_Bottom.vi"("error in"=w177, "vi 2 ref"=w176, "vi 1 ref"=w179) -> ("error out"=w169:errorcluster, "vi 2 ref dup"=w175:refnum<vi>, "vi 1 ref dup"=w178:refnum<vi>)  [unwired: 6 in]
        n65 = To Variant(anything=w181) -> (Variant=w180:variant)
        n66 = Build Array (concatenate)(w184, w180) -> (w183:variant[])
        n67 = Close Reference(reference=w175, error in (no error)=w169) -> (error out=w168:errorcluster)
        n68 = call "GenINI_Create_Constants.vi"("error in"=w168, "Data array"=w183, "Terminal names"=w185, "vi ref"=w178) -> ("error out"=w174:errorcluster, "vi ref dup"=w171:refnum<vi>)  [unwired: 6 in]
        n69 = call "GenINI_Wire_Terminal.vi"("error in"=w174, "Terminal  name"="value", "Wire source ref"=w173, "vi ref"=w171) -> ("error out"=w167:errorcluster, "Wire source ref dup"=w166:refnum<vi>, "vi ref dup"=w170:refnum<vi>)  [unwired: 5 in]
        n70 = stacked-sequence {
          tunnel: w166 -> [_]
          frame #0 {
            # "Will close wire source ref\nafter for loop."
          }
        }
      }
      frame #2 {
        w214 = string[] ["section", "key", "default value"]  # Terminal names
        w222 = refnum<vi> refnum  # PolymorphicSubVI
        # "Last VI in drop line"
        # "Last VI in drop line"
        # "Current Bundle by name terminal ref."
        # "Drop key read"
        # "Create BD constants"
        n71 = New VI Object(vi object class=w222, owner refnum=w217, position/next to=w216, 6:w215, 8:w218) -> (object refnum=w221:refnum<vi>, 0:w219:errorcluster)  [unwired: 3 in]
        n72 = property class="PolySubVI"(reference=w221, error in=w219, "SelectedType"=2 ("Selected Type")) -> (reference out=w208:refnum<vi>, error out=w206:errorcluster)
        n73 = Decimal String To Number(string=w211, default (0L)=0 ("default (0 I32)")) -> (number=w210:i32)  [unwired: 1 in, 1 out]
        n74 = call "GenINI_Wire_Top_And_Bottom.vi"("error in"=w206, "vi 2 ref"=w205, "vi 1 ref"=w208) -> ("error out"=w198:errorcluster, "vi 2 ref dup"=w204:refnum<vi>, "vi 1 ref dup"=w207:refnum<vi>)  [unwired: 6 in]
        n75 = To Variant(anything=w210) -> (Variant=w209:variant)
        n76 = Build Array (concatenate)(w213, w209) -> (w212:variant[])
        n77 = Close Reference(reference=w204, error in (no error)=w198) -> (error out=w197:errorcluster)
        n78 = call "GenINI_Create_Constants.vi"("error in"=w197, "Data array"=w212, "Terminal names"=w214, "vi ref"=w207) -> ("error out"=w203:errorcluster, "vi ref dup"=w200:refnum<vi>)  [unwired: 6 in]
        n79 = call "GenINI_Wire_Terminal.vi"("error in"=w203, "Terminal  name"="value", "Wire source ref"=w202, "vi ref"=w200) -> ("error out"=w196:errorcluster, "Wire source ref dup"=w195:refnum<vi>, "vi ref dup"=w199:refnum<vi>)  [unwired: 5 in]
        n80 = stacked-sequence {
          tunnel: w195 -> [_]
          frame #0 {
            # "Will close wire source ref\nafter for loop."
          }
        }
      }
      frame #3 {
        w242 = string[] ["section", "key", "default value"]  # Terminal names
        w250 = refnum<vi> refnum  # PolymorphicSubVI
        # "String to path is sketchy here, but will do."
        # "Last VI in drop line"
        # "Last VI in drop line"
        # "Current Bundle by name terminal ref."
        # "Drop key read"
        # "Create BD constants"
        n81 = New VI Object(vi object class=w250, owner refnum=w245, position/next to=w244, 6:w243, 8:w246) -> (object refnum=w249:refnum<vi>, 0:w247:errorcluster)  [unwired: 3 in]
        n82 = property class="PolySubVI"(reference=w249, error in=w247, "SelectedType"=3 ("Selected Type")) -> (reference out=w239:refnum<vi>, error out=w237:errorcluster)
        n83 = String To Path(string=w225) -> (path=w224:path)
        n84 = To Variant(anything=w224) -> (Variant=w223:variant)
        n85 = call "GenINI_Wire_Top_And_Bottom.vi"("error in"=w237, "vi 2 ref"=w236, "vi 1 ref"=w239) -> ("error out"=w229:errorcluster, "vi 2 ref dup"=w235:refnum<vi>, "vi 1 ref dup"=w238:refnum<vi>)  [unwired: 6 in]
        n86 = Build Array (concatenate)(w241, w223) -> (w240:variant[])
        n87 = Close Reference(reference=w235, error in (no error)=w229) -> (error out=w228:errorcluster)
        n88 = call "GenINI_Create_Constants.vi"("error in"=w228, "Data array"=w240, "Terminal names"=w242, "vi ref"=w238) -> ("error out"=w234:errorcluster, "vi ref dup"=w231:refnum<vi>)  [unwired: 6 in]
        n89 = call "GenINI_Wire_Terminal.vi"("error in"=w234, "Terminal  name"="value", "Wire source ref"=w233, "vi ref"=w231) -> ("error out"=w227:errorcluster, "Wire source ref dup"=w226:refnum<vi>, "vi ref dup"=w230:refnum<vi>)  [unwired: 5 in]
        n90 = stacked-sequence {
          tunnel: w226 -> [_]
          frame #0 {
            # "Will close wire source ref\nafter for loop."
          }
        }
      }
      frame #4 {
        w271 = string[] ["section", "key", "default value", "read raw string? (F)"]  # Terminal names
        w279 = refnum<vi> refnum  # PolymorphicSubVI
        # "Last VI in drop line"
        # "Last VI in drop line"
        # "Current Bundle by name terminal ref."
        # "Drop key read"
        # "Create BD constants"
        n91 = New VI Object(vi object class=w279, owner refnum=w274, position/next to=w273, 6:w272, 8:w275) -> (object refnum=w278:refnum<vi>, 0:w276:errorcluster)  [unwired: 3 in]
        n92 = property class="PolySubVI"(reference=w278, error in=w276, "SelectedType"=4 ("Selected Type")) -> (reference out=w267:refnum<vi>, error out=w265:errorcluster)
        n93 = To Variant(anything=w253) -> (Variant=w268:variant)
        n94 = To Variant(anything=w252) -> (Variant=w251:variant)
        n95 = call "GenINI_Wire_Top_And_Bottom.vi"("error in"=w265, "vi 2 ref"=w264, "vi 1 ref"=w267) -> ("error out"=w257:errorcluster, "vi 2 ref dup"=w263:refnum<vi>, "vi 1 ref dup"=w266:refnum<vi>)  [unwired: 6 in]
        n96 = Build Array (concatenate)(w270, w268, w251) -> (w269:variant[])
        n97 = Close Reference(reference=w263, error in (no error)=w257) -> (error out=w256:errorcluster)
        n98 = call "GenINI_Create_Constants.vi"("error in"=w256, "Data array"=w269, "Terminal names"=w271, "vi ref"=w266) -> ("error out"=w262:errorcluster, "vi ref dup"=w259:refnum<vi>)  [unwired: 6 in]
        n99 = call "GenINI_Wire_Terminal.vi"("error in"=w262, "Terminal  name"="value", "Wire source ref"=w261, "vi ref"=w259) -> ("error out"=w255:errorcluster, "Wire source ref dup"=w254:refnum<vi>, "vi ref dup"=w258:refnum<vi>)  [unwired: 5 in]
        n100 = stacked-sequence {
          tunnel: w254 -> [_]
          frame #0 {
            # "Will close wire source ref\nafter for loop."
          }
        }
      }
      frame #5 {
        w300 = string[] ["section", "key", "default value"]  # Terminal names
        w308 = refnum<vi> refnum  # PolymorphicSubVI
        # "Last VI in drop line"
        # "Last VI in drop line"
        # "Current Bundle by name terminal ref."
        # "Drop key read"
        # "Create BD constants"
        n101 = New VI Object(vi object class=w308, owner refnum=w303, position/next to=w302, 6:w301, 8:w304) -> (object refnum=w307:refnum<vi>, 0:w305:errorcluster)  [unwired: 3 in]
        n102 = property class="PolySubVI"(reference=w307, error in=w305, "SelectedType"=5 ("Selected Type")) -> (reference out=w294:refnum<vi>, error out=w292:errorcluster)
        n103 = Decimal String To Number(string=w297, default (0L)=u32 0 ("default (0 I32)")) -> (number=w296:u32)  [unwired: 1 in, 1 out]
        n104 = call "GenINI_Wire_Top_And_Bottom.vi"("error in"=w292, "vi 2 ref"=w291, "vi 1 ref"=w294) -> ("error out"=w284:errorcluster, "vi 2 ref dup"=w290:refnum<vi>, "vi 1 ref dup"=w293:refnum<vi>)  [unwired: 6 in]
        n105 = To Variant(anything=w296) -> (Variant=w295:variant)
        n106 = Build Array (concatenate)(w299, w295) -> (w298:variant[])
        n107 = Close Reference(reference=w290, error in (no error)=w284) -> (error out=w283:errorcluster)
        n108 = call "GenINI_Create_Constants.vi"("error in"=w283, "Data array"=w298, "Terminal names"=w300, "vi ref"=w293) -> ("error out"=w289:errorcluster, "vi ref dup"=w286:refnum<vi>)  [unwired: 6 in]
        n109 = call "GenINI_Wire_Terminal.vi"("error in"=w289, "Terminal  name"="value", "Wire source ref"=w288, "vi ref"=w286) -> ("error out"=w282:errorcluster, "Wire source ref dup"=w281:refnum<vi>, "vi ref dup"=w285:refnum<vi>)  [unwired: 5 in]
        n110 = stacked-sequence {
          tunnel: w281 -> [_]
          frame #0 {
            # "Will close wire source ref\nafter for loop."
          }
        }
      }
    }
  }
  n111 = Close Reference(reference=w39, error in (no error)=w41) -> (error out=w40:errorcluster)
  n112 = Open VI Object Reference(7:w87, 8:w40, 10:"Close Config Data.vi" ("name/order"), 11:w18) -> (0:w34:errorcluster, 3:w36:refnum<vi>)
  n113 = call "GenINI_Wire_Top_And_Bottom.vi"("error in"=w34, "vi 2 ref"=w35, "vi 1 ref"=w36) -> ("error out"=w31:errorcluster, "vi 2 ref dup"=w32:refnum<vi>, "vi 1 ref dup"=w33:refnum<vi>)  [unwired: 6 in]
  n114 = Close Reference(reference=w33, error in (no error)=w31) -> (error out=w71:errorcluster)
  n115 = Close Reference(reference=w32, error in (no error)=w71) -> (error out=w63:errorcluster)
  n116 = property class="VI"(reference=w18, error in=w63, "BD Win.Origin"=T4 {"Horizontal"=0, "Vertical"=0} ("Block Diagram Window:Origin")) -> (reference out=w75:refnum<vi>, error out=w74:errorcluster)
  n117 = invoke class="VI" method="BD.CleanUp"(reference=w75, error in=w74) -> (reference out=w4:refnum<vi>, error out=w2:errorcluster)  [unwired: 1 in, 1 out]
  n118 = invoke class="VI" method="Save.Instrument"(reference=w4, error in=w2, "Path to saved file"=w5) -> (reference out=w3:refnum<vi>, error out=w1:errorcluster)  [unwired: 3 in, 4 out]
  n119 = Close Reference(reference=w3, error in (no error)=w1) -> (error out=→"error out":errorcluster)
  "INI read values dup" <- "INI read values"
  "Typedef path dup" <- "Typedef path"
